vi "ReadConfiguredPower.vi"(0 "VISA resource name":refnum<visa-resource-name>, 11 "error in (no error)":errorcluster) -> (2 "RF Power ?(T: On)":bool=TRUE, 4 "VISA resource name out":refnum<visa-resource-name>, 15 "error out":errorcluster)   [LabVIEW 2018, in "Keysight PNA Series.lvlib"]
doc: "Configures the RF power."
uses:
  Keysight PNA Series.lvlib
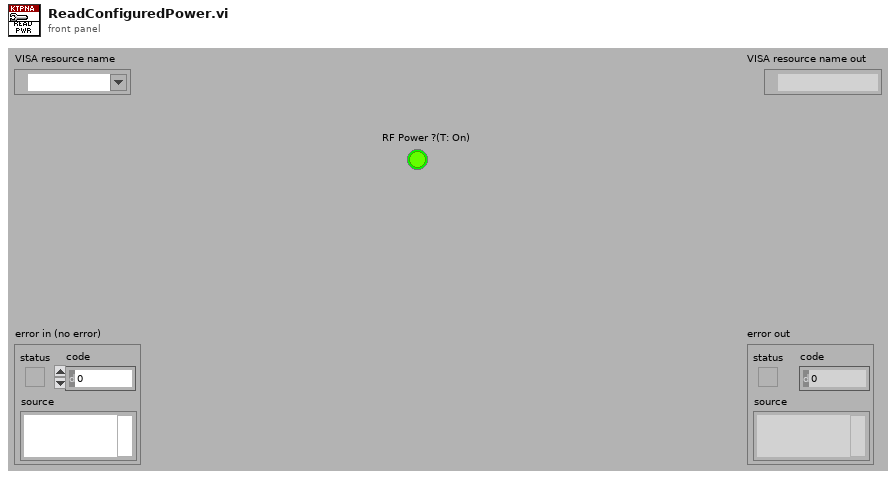
[diagram p1: front panel]
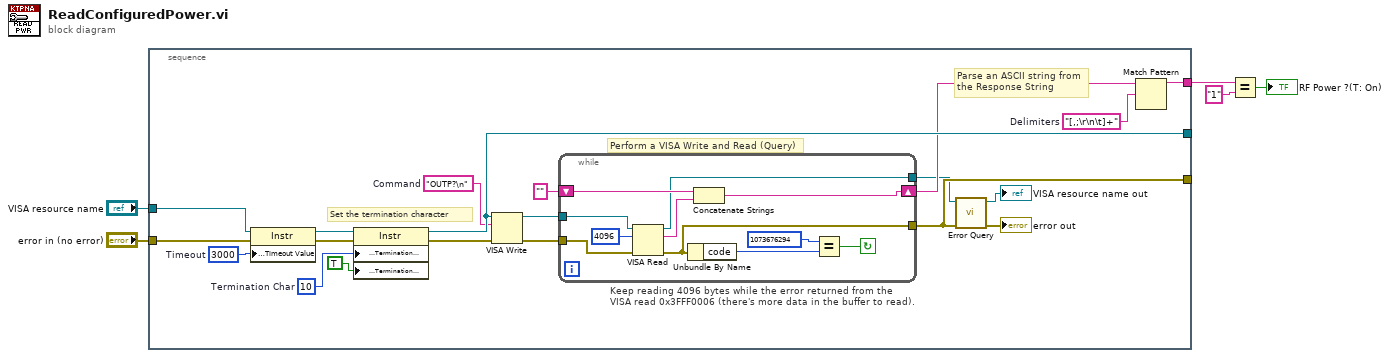
[diagram p0: block diagram]
diagram:
  n1 = stacked-sequence {
    tunnel: "VISA resource name" -> [w12]
    tunnel: "error in (no error)" -> [w11]
    tunnel: [w25] -> _
    tunnel: [w22] -> w4
    tunnel: [w7] -> _
    frame #0 {
      w23 = "[,;\r\n\t]+"  # Delimiters
      w21 = "OUTP?\n"  # Command
      w15 = u8 10  # Termination Char
      w10 = u32 3000  # Timeout
      # "Parse an ASCII string from the Response String"
      # "Perform a VISA Write and Read (Query)"
      # "Keep reading 4096 bytes while the error returned from the\nVISA read 0x3FFF0006 (there's more data in the buffer to read)."
      # "Set the termination character"
      n2 = property class="Instr"(reference=w12, error in=w11, "General Settings:Timeout Value"=w10) -> (reference out=w16:refnum<visa-resource-name>, error out=w13:errorcluster)
      n3 = property class="Instr"(reference=w16, error in=w13, "Message Based Settings:Termination Character"=w15, "Message Based Settings:Termination Character Enable"=TRUE ("enable")) -> (reference out=w25:refnum<visa-resource-name>, error out=w14:errorcluster)
      n4 = VISA Write(VISA resource name=w25, write buffer=w21, error in (no error)=w14) -> (VISA resource name out=w18:refnum<visa-resource-name>, error out=w19:errorcluster)  [unwired: 1 out]
      n5 = while {
        tunnel: w18 -> [w33]
        shift-right: [w27] -> w24
        shift-left: "" -> [w32]
        tunnel: w19 -> [w30]
        tunnel: [w29] -> w7
        tunnel: [w26] -> w6
        stop <- w28 continue-if-true
        n6 = VISA Read(VISA resource name=w33, byte count=u32 4096 ("byte count (0)"), error in (no error)=w30) -> (VISA resource name out=w26:refnum<visa-resource-name>, read buffer=w31:string, error out=w29:errorcluster)  [unwired: 1 out]
        n7 = Unbundle By Name(w29) -> ("code"=w35:i32)
        n8 = Concatenate Strings(w32, w31) -> (w27:string)
        n9 = Equal?(x=1073676294, y=w35) -> (x = y?=w28:bool)
      }
      n10 = call "Error Query.vi"("error in (no error)"=w7, "VISA resource name"=w6) -> ("error out"=→"error out":errorcluster, "VISA resource name out"=→"VISA resource name out":refnum<visa-resource-name>)  [unwired: 6 in, 2 out]
      n11 = Match Pattern(string=w24, regular expression=w23) -> (before substring=w22:string)  [unwired: 4 out]
    }
  }
  n12 = Equal?(x=w4, y="1") -> (x = y?=→"RF Power ?(T: On)":bool)
